vi "Action.vi"(8 "error in (no error)":errorcluster, 10 "Actor in":refnum<class "Tamagotchi Basic Actor.lvclass">, 11 "Clean Message in":refnum<class "Clean Message.lvclass">) -> (0 "error out":errorcluster, 2 "Actor out":refnum<class "Tamagotchi Basic Actor.lvclass">, 3 "Clean Message out":refnum<class "Clean Message.lvclass">)   [LabVIEW 2026, in "Clean Message.lvclass"]
uses:
  Clean Message.lvclass
  Tamagotchi Basic Actor/Tamagotchi Basic Actor.lvclass
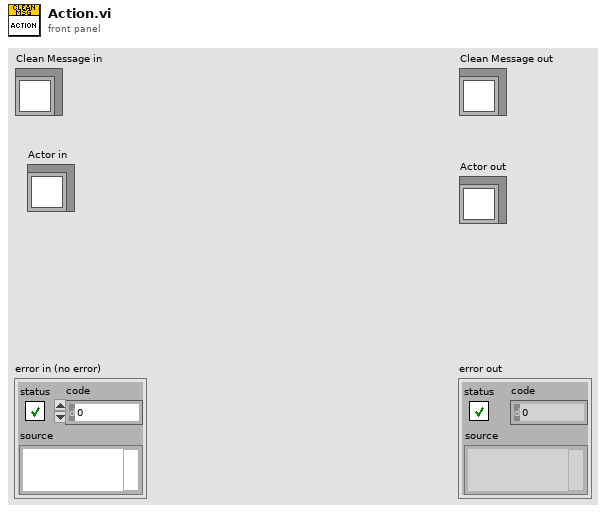
[diagram p1: front panel]
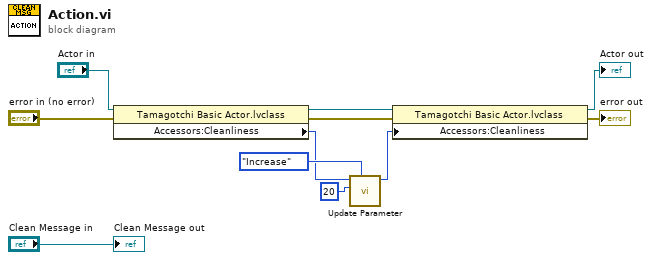
[diagram p0: block diagram]
diagram:
  n1 = property class="Tamagotchi Basic Actor.lvclass"(reference="Actor in", error in="error in (no error)") -> (reference out=w8:refnum<class "Tamagotchi Basic Actor.lvclass">, error out=w2:errorcluster, "Accessors:Cleanliness"=w9:i16)
  n2 = call "Update Parameter.vi"("Action"=enum16{"Increase", "Decrease"}."Increase", "Modifier"=i16 20 ("y"), "Parameter"=w9) -> ("New Value"=w7:i16)  [unwired: 8 in]
  n3 = property class="Tamagotchi Basic Actor.lvclass"(reference=w8, error in=w2, "Accessors:Cleanliness"=w7) -> (reference out=→"Actor out":refnum<class "Tamagotchi Basic Actor.lvclass">, error out=→"error out":errorcluster)
  "Clean Message out" <- "Clean Message in"
